vi "Stalker.vi"(8 "Error In":errorcluster, 11 "Refnum's In":T1={"Gyro"="Gyro", "Mtr 1"="LeftMtr", "Mtr 2"="RightMtr"}) -> (0 "Error Out":errorcluster, 3 "Refnum's Out":T1={"Gyro"="Gyro", "Mtr 1"="LeftMtr", "Mtr 2"="RightMtr"})   [LabVIEW 2016]
uses:
  Robot Global Data.vi
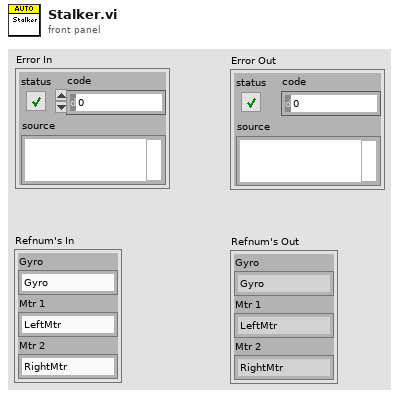
[diagram p1: front panel]
types:
  T1 = cluster{"Gyro":string, "Mtr 1":string, "Mtr 2":string}
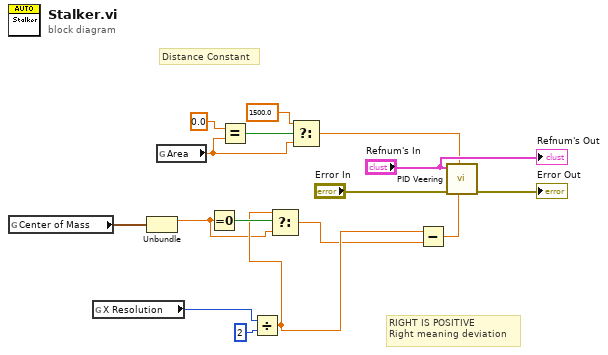
[diagram p0: block diagram]
diagram:
  # "Distance Constant"
  # "RIGHT IS POSITIVE\nRight meaning deviation"
  n1 = global read "Robot Global Data.vi" "Center of Mass"() -> (w14:cluster{"X":dbl, "Y":dbl})
  n2 = global read "Robot Global Data.vi" "X Resolution"() -> (w12:i32)
  n3 = Unbundle(w14) -> ("X"=w2:dbl)  [unwired: 1 out]
  n4 = global read "Robot Global Data.vi" "Area"() -> (w7:dbl)
  n5 = Equal To 0?(x=w2) -> (x = 0?=w4:bool)
  n6 = Equal?(x=0.0 ("y"), y=w7) -> (x = y?=w10:bool)
  n7 = Divide(x=w12, y=2) -> (x/y=w3:dbl)
  n8 = Select(t=w3, s=w4, f=w2) -> (s? t:f=w1:dbl)
  n9 = Select(t=1500.0 ("x"), s=w10, f=w7) -> (s? t:f=w6:dbl)
  n10 = Subtract(x=w3, y=w1) -> (x-y=w5:dbl)
  n11 = call "PID Veering.vi"("Deviation"=w5, "Current Distance"=w6, "error in (no error)"="Error In", "Refnum's"="Refnum's In") -> ("error out"=→"Error Out":errorcluster)  [unwired: 7 in]
  "Refnum's Out" <- "Refnum's In"
